vi "two_button.vi"(7 "callee":refnum<vi>, 8 "error in (no error)":errorcluster, 10 "configuration":T2, 11 "v1 in":refnum<class "v1.lvclass">) -> (0 "error out":errorcluster, 2 "dialog_selection":T1, 3 "v1 out":refnum<class "v1.lvclass">)   [LabVIEW 2015, in "lv-dialog-interfaces.lvlib" / "v1.lvlib" / "v1.lvclass"]
uses:
  v1.lvclass
  <userlib>/antonio-alexander/lv-dialog/api/v1/public/_controls/selection.ctl
  lv-dialog-interfaces.lvlib
  <userlib>/antonio-alexander/lv-dialog/api/v1/v1.lvlib
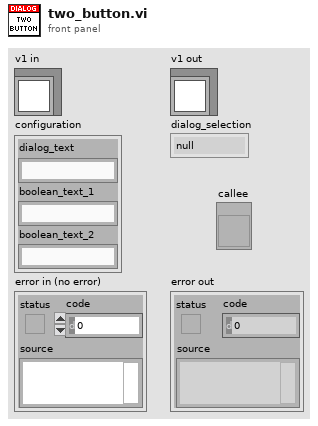
[diagram p1: front panel]
types:
  T1 = typedef "lv-dialog.lvlib/v1.lvlib/selection.ctl" = enum16{"null", "panel_closed", "button_1", "button_2", "button_3", "cancelled"}
  T2 = cluster{"dialog_text":string, "boolean_text_1":string, "boolean_text_2":string}
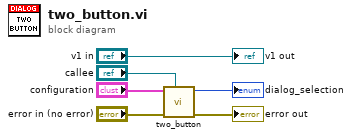
[diagram p0: block diagram]
diagram:
  n1 = call "two_button.vi"("callee"="callee", "error in (no error)"="error in (no error)", "configuration"="configuration") -> ("error out"=→"error out":errorcluster, "dialog_selection"=→"dialog_selection":T1)  [unwired: 7 in]
  "v1 out" <- "v1 in"
